vi "DriveDistanceY.vi"(2 "Parameter String":string, 3 "Reinit":bool) -> (0 "Error Out":errorcluster, 1 "Increment":bool)   [LabVIEW 2019]
doc: "The swerve drive base will translate in the field-centric Y direction at a speed specified by the joystick command. This is a \"dumb\" algorithm, there is no feedback controller and the direction of translation must be specified manually. Any complex or critical translations should be handled using either the Path Follower or auto-targeting. \n\nParameters:\n1. relative travel distance in the field-centric Y direction --> (in) [0,315]\n2. relative translation speed --> [-1,1]"
uses:
  SafeParser_Float.vi
  dsinstructions.vi
  sensors.vi
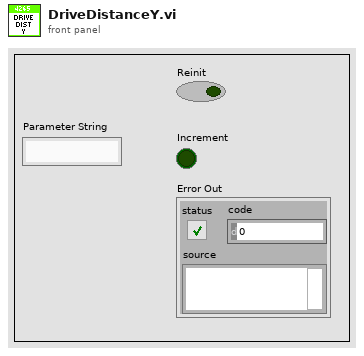
[diagram p1: front panel]
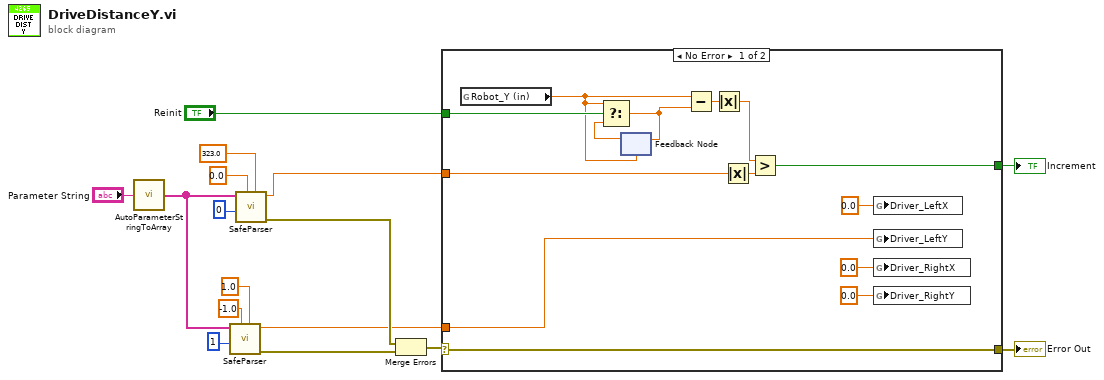
[diagram p0: block diagram]
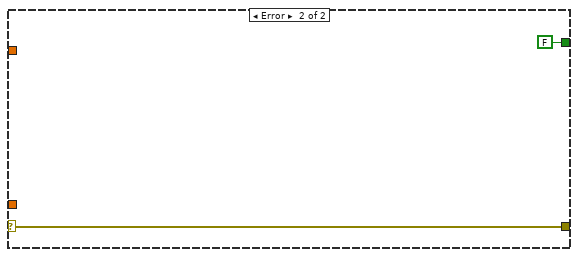
[diagram p2: hidden frame]
diagram:
  n1 = call "AutoParameterStringToArray.vi"("Parameter String"="Parameter String") -> ("Parsed Parameters"=w9:string[])
  n2 = call-poly "SafeParser.vi"("Maximum"=1.0, "Minimum"=-1.0, "Array Index"=1 ("Parameter Index"), "String Array"=w9) -> ("Error Out"=w7:errorcluster, "Typecast  Value"=w3:dbl)  [unwired: 6 in]
  n3 = call-poly "SafeParser.vi"("Maximum"=323.0, "Minimum"=0.0, "Array Index"=0 ("Parameter Index"), "String Array"=w9) -> ("Error Out"=w5:errorcluster, "Typecast  Value"=w4:dbl)  [unwired: 6 in]
  n4 = Merge Errors(w5, w7) -> (w6:errorcluster)
  n5 = case shown="No Error" w6 {
    selector: w6 -> [w20 w32]
    tunnel: [w30 FALSE] -> w16
    tunnel: "Reinit" -> [w28 _]
    tunnel: [w20 w32] -> w14
    tunnel: w4 -> [w19 _]
    tunnel: w3 -> [w18 _]
    frame No Error {
      n6 = global read "sensors.vi" "Robot_Y (in)"() -> (w27:dbl)
      n7 = feedback #1(w27) -> (w29:dbl)
      n8 = Select(t=w27, s=w28, f=w29) -> (s? t:f=w26:dbl)
      n9 = feedback-in #1(w26) -> ()
      n10 = Subtract(x=w27, y=w26) -> (x-y=w25:dbl)
      n11 = Absolute Value(x=w25) -> (abs(x)=w22:dbl)
      n12 = Absolute Value(x=w19) -> (abs(x)=w21:dbl)
      n13 = Greater?(x=w22, y=w21) -> (0:w30:bool)
      n14 = global write "dsinstructions.vi" "Driver_LeftX"(0.0 ("Driver_LeftX")) -> ()
      n15 = global write "dsinstructions.vi" "Driver_LeftY"(w18) -> ()
      n16 = global write "dsinstructions.vi" "Driver_RightX"(0.0 ("Driver_RightX")) -> ()
      n17 = global write "dsinstructions.vi" "Driver_RightY"(0.0 ("Driver_RightX")) -> ()
    }
    frame Error {
    }
  }
  "Increment" <- w16
  "Error Out" <- w14
